vi "Logout Role.vi"(8 "error in (no error)":errorcluster, 11 "Role Manager in":refnum<class "Role Manager.lvclass">) -> (0 "error out":errorcluster, 3 "Role Manager out":refnum<class "Role Manager.lvclass">)   [LabVIEW 2020, in "Volatus.lvlib" / "Role Manager.lvclass"]
uses:
  Role Manager.lvclass
  C:/dev/lv20CE/relink/lv-volatus/Volatus/Module/Module.lvclass
  Module/Module.lvclass/Module.ctl
  Role Manager.lvclass/Role Manager.ctl
  Roles API/Roles API.lvclass
  Module/Module.lvclass
  C:/dev/lv20CE/relink/lv-volatus/Volatus/Role Manager/Role Manager.lvclass
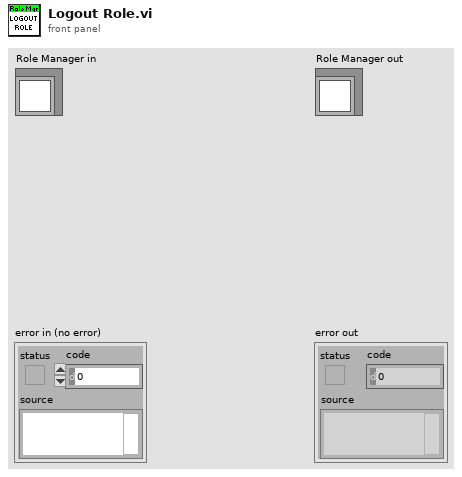
[diagram p1: front panel]
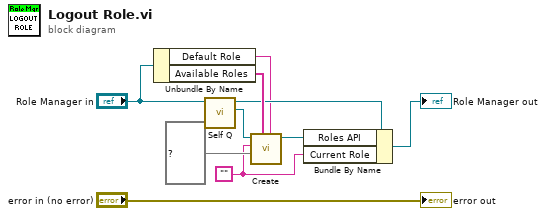
[diagram p0: block diagram]
diagram:
  w3 = ""
  n1 = Unbundle By Name("Role Manager in") -> ("Default Role"=w1:string, "Available Roles"=w9:string[])
  n2 = call "Self Q.vi"("Module in"="Role Manager in") -> ("Self Q"=w8:refnum<class "MessageQ.lvclass">, "Module out"=w7:refnum<class "Role Manager.lvclass">)  [unwired: 9 in]
  n3 = call "Create.vi"("Default Role"=w1, "Available"=w9, "Effective Roles"=set{string} {}, "Current Role"=w3, "Manager"=w8) -> ("Roles API out"=w6:refnum<class "Roles API.lvclass">)  [unwired: 5 in, 1 out]
  n4 = Bundle By Name(cluster=w7, "Roles API"=w6, "Current Role"=w3) -> (→"Role Manager out":refnum<class "Role Manager.lvclass">)
  "error out" <- "error in (no error)"
